vi "Read Sine Grap to binary file.vi"() -> ()   [LabVIEW 2020]
panel:
  out "Waveform Graph":dbl[](graph)
  in  "Path":path
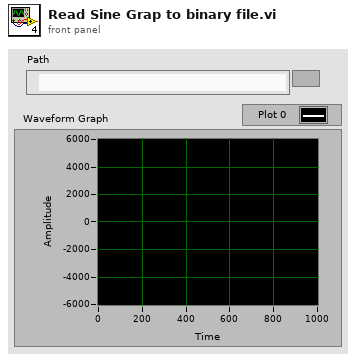
[diagram p1: front panel]
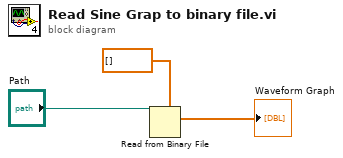
[diagram p0: block diagram]
diagram:
  n1 = Read from Binary File(5:dbl[] [], 11:"Path") -> (2:→"Waveform Graph":dbl[])  [unwired: 4 in, 3 out]
